vi "WriteFpgaData.vi"(0 "Stand":refnum<class "Stand.lvclass">, 11 "error in (no error)":errorcluster) -> (4 "Stand out":refnum<class "Stand.lvclass">, 15 "error out":errorcluster)   [LabVIEW 2019, in "Stand.lvclass"]
uses:
  Stand.lvclass
  Stand.lvclass/Stand.ctl
  Sig_AO_class/Sig_AO.lvclass/Sig_AO.ctl
  Sig_DO_Simple_class/Sig_DO_Simple.lvclass/Sig_DO_Simple.ctl
  FPGA_Interface_class/FPGA_Interface.lvclass
  Sig_DO_Simple_class/Sig_DO_Simple.lvclass
  Sig_AO_class/Sig_AO.lvclass
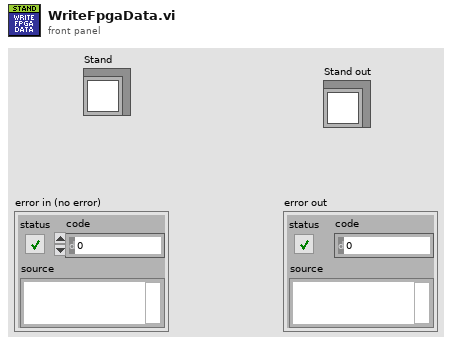
[diagram p1: front panel]
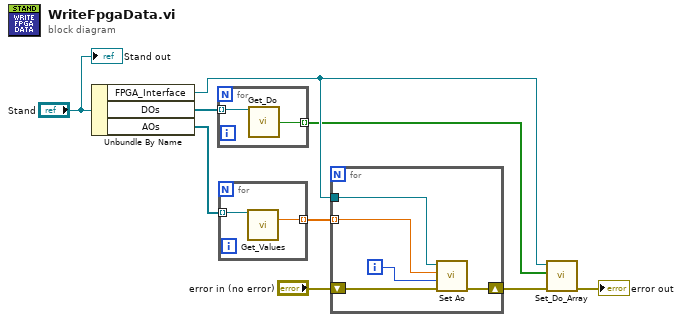
[diagram p0: block diagram]
diagram:
  n1 = Unbundle By Name("Stand") -> ("FPGA_Interface"=w3:refnum<class "FPGA_Interface.lvclass">, "DOs"=w8:refnum<class "Sig_DO_Simple.lvclass">[], "AOs"=w7:refnum<class "Sig_AO.lvclass">[])
  n2 = for {
    tunnel: w8 -> [w11] mode=indexing
    tunnel: [w10] -> w2 mode=indexing
    n3 = call "Get_Do.vi"("reference in"=w11) -> ("DO"=w10:bool)  [unwired: 14 in]
  }
  n4 = for {
    tunnel: w7 -> [w13] mode=indexing
    tunnel: [w12] -> w6 mode=indexing
    n5 = call "Get_Values.vi"("reference in"=w13) -> ("AO"=w12:dbl)  [unwired: 14 in]
  }
  n6 = for {
    tunnel: w6 -> [w18] mode=indexing
    shift-right: [w16] -> w4
    shift-left: "error in (no error)" -> [w15]
    tunnel: w3 -> [w14]
    i -> [w17]
    n7 = call-dynamic "Set Ao.vi"("error in (no error)"=w15, "Indx"=w17, "Value"=w18, "FPGA_Interface in"=w14) -> ("error out"=w16:errorcluster)  [unwired: 6 in, 1 out]
  }
  n8 = call-dynamic "Set_Do_Array.vi"("error in (no error)"=w4, "DOs"=w2, "reference in"=w3) -> ("error out"=→"error out":errorcluster)  [unwired: 7 in, 1 out]
  "Stand out" <- "Stand"
